vi "Write Solvent Table.vi"(8 "Error In":errorcluster, 10 "Layer Information Array In":T1 {"Deposition Method" items=["Front Electrode", "Electron Transport Layer", "Active Layer", "Hole Transport Layer", "Back Electrode", "Custom Layer"]; "Layer Type" items=["Front Electrode", "Electron Transport Layer", "Active Layer", "Hole Transport Layer", "Back Electrode", "Custom Layer"]}, 11 "Database Full Information In":T2 {"Database Write Information"."Layer Information Array"."Deposition Method" items=["Blade Coating", "Spin Coating", "Thermal Evaporation", "E-Beam Evaporation", "Sputtering", "Drop Casting", "Dip Coating", "Pulsed Laser Deposition", "Chemival Vapour Deposition", "Atomic Layer Deposition", "Spray Coating", "Screen Printing", "Electroplating", "Molecular Beam Epitaxy", "Custom Deposition"]; "Database Write Information"."Layer Information Array"."Layer Type" items=["Front Electrode", "Electron Transport Layer", "Active Layer", "Hole Transport Layer", "Back Electrode", "Custom Layer"]}) -> (0 "Error Out":errorcluster, 3 "Database Full Information Out":T2 {"Database Write Information"."Layer Information Array"."Deposition Method" items=["Blade Coating", "Spin Coating", "Thermal Evaporation", "E-Beam Evaporation", "Sputtering", "Drop Casting", "Dip Coating", "Pulsed Laser Deposition", "Chemival Vapour Deposition", "Atomic Layer Deposition", "Spray Coating", "Screen Printing", "Electroplating", "Molecular Beam Epitaxy", "Custom Deposition"]; "Database Write Information"."Layer Information Array"."Layer Type" items=["Front Electrode", "Electron Transport Layer", "Active Layer", "Hole Transport Layer", "Back Electrode", "Custom Layer"]})   [LabVIEW 2020]
uses:
  Data Clusters/Database Information.ctl
  Data Clusters/Layer Information Cluster.ctl
  <vilib>/addons/database/Connection.llb/Conn ObjectReference.ctl
  <vilib>/addons/database/NI_Database_API.lvlib
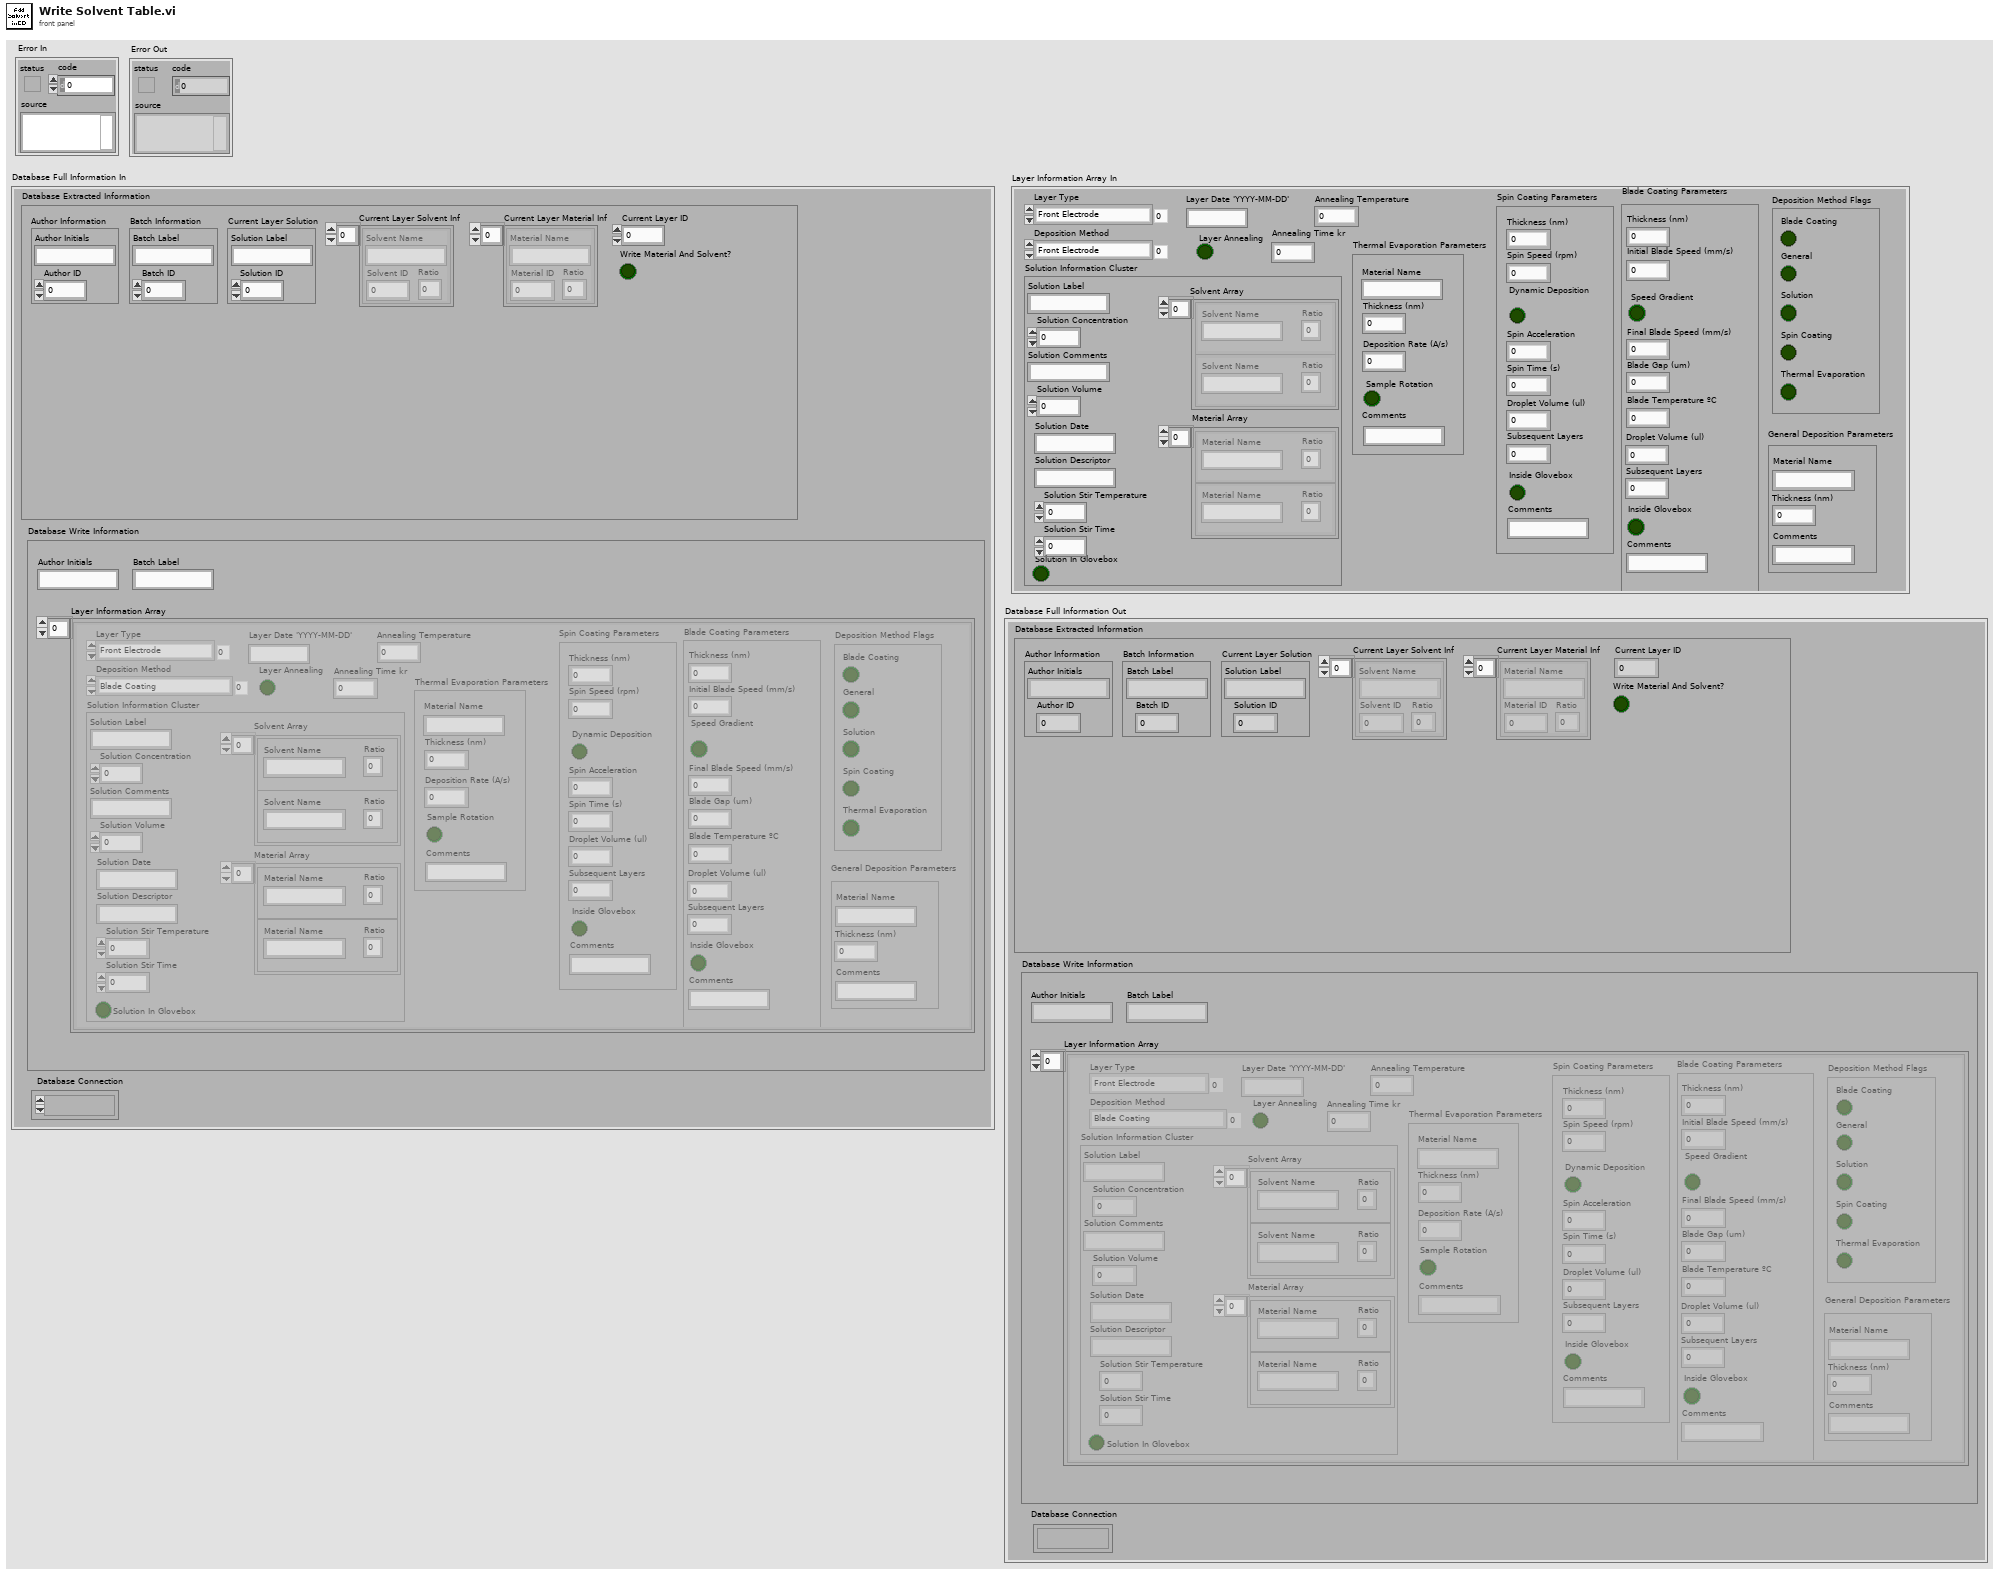
[diagram p1: front panel]
types:
  T1 = typedef "Layer Information Cluster.ctl" = cluster{"Solution Information Cluster":cluster{"Solution Label":string, "Solution Concentration":dbl, "Solution Comments ":string, "Solution Volume ":dbl, "Solution Date ":string, "Solution Descriptor ":string, "Solution Stir Temperature ":dbl, "Solution Stir Time ":dbl, "Solution In Glovebox":bool, "Solvent Array":cluster{"Solvent Name":string, "Ratio":dbl}[], "Material Array":cluster{"Material Name":string, "Ratio":dbl}[]}, "Layer Type":u16, "Deposition Method":u16, "Layer Annealing":bool, "General Deposition Parameters":cluster{"Thickness (nm)":dbl, "Comments":string, "Material Name":string}, "Blade Coating Parameters":cluster{"Thickness (nm)":dbl, "Initial Blade Speed (mm/s)":dbl, "Speed Gradient":bool, "Final Blade Speed (mm/s)":dbl, "Blade Gap (um)":dbl, "Droplet Volume (ul)":dbl, "Subsequent Layers":dbl, "Inside Glovebox":bool, "Comments":string, "Blade Temperature ºC":dbl}, "Spin Coating Parameters":cluster{"Thickness (nm)":dbl, "Spin Speed (rpm)":dbl, "Dynamic Deposition":bool, "Spin Acceleration":dbl, "Spin Time (s)":dbl, "Droplet Volume (ul)":dbl, "Subsequent Layers":dbl, "Inside Glovebox":bool, "Comments":string}, "Thermal Evaporation Parameters":cluster{"Deposition Rate (A/s)":dbl, "Thickness (nm)":dbl, "Comments":string, "Material Name":string, "Sample Rotation":bool}, "Layer Date 'YYYY-MM-DD'":string, "Annealing Time kr":dbl, "Annealing Temperature":dbl, "Deposition Method Flags":cluster{"Blade Coating":bool, "General ":bool, "Solution":bool, "Spin Coating":bool, "Thermal Evaporation":bool}}
  T2 = typedef "Database Information.ctl" = cluster{"Database Extracted Information":cluster{"Author Information":cluster{"Author Initials":string, "Author ID":i32}, "Batch Information":cluster{"Batch Label":string, "Batch ID":i32}, "Current Layer Solution":cluster{"Solution Label":string, "Solution ID":i32}, "Current Layer ID":i32, "Current Layer Solvent Inf":cluster{"Solvent Name":string, "Solvent ID":i32, "Ratio":dbl}[], "Current Layer Material Inf":cluster{"Material Name":string, "Material ID":i32, "Ratio":dbl}[], "Write Material And Solvent?":bool}, "Database Write Information":cluster{"Author Initials":string, "Batch Label":string, "Layer Information Array":T1[]}, "Database Connection":T3}
  T3 = typedef "NI_Database_API.lvlib/Conn ObjectReference.ctl" = refnum<k1>
  T4 = cluster{"Solvent Name":string, "Solvent ID":i32, "Ratio":dbl}
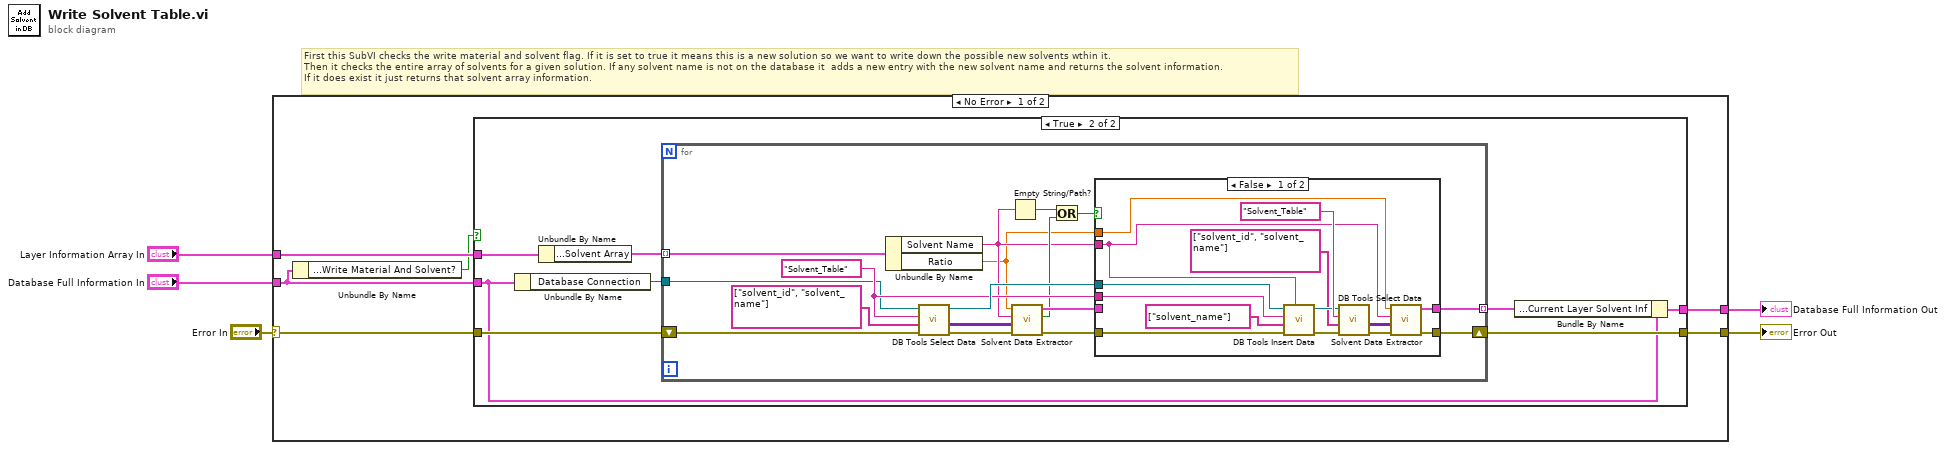
[diagram p0: block diagram]
diagram:
  # "First this SubVI checks the write material and solvent flag. If it is set to true it means this is a new solution so we want to write down the possible new solvents wthin it.\nThen it checks the entire array of solvents for a given solution. If any solvent name is not on the database it  adds a new entry with the new solvent name and returns the solvent information.\nIf it does exist it just returns that solvent array information."
  n1 = case shown="No Error" "Error In" {
    selector: "Error In" -> [w11 w56]
    tunnel: [w10 w56] -> w3
    tunnel: "Database Full Information In" -> [w7 w55]
    tunnel: [w9 w55] -> w2
    tunnel: "Layer Information Array In" -> [w8 _]
    frame No Error {
      n2 = Unbundle By Name(w7) -> ("Database Extracted Information.Write Material And Solvent?"=w6:bool)
      n3 = case shown="True" w6 {
        tunnel: w11 -> [w12 w21]
        tunnel: [w12 w20] -> w10
        tunnel: w7 -> [w13 w19]
        tunnel: [w13 w17] -> w9
        tunnel: w8 -> [_ w15]
        frame False {
        }
        frame True {
          n4 = Unbundle By Name(w19) -> ("Database Connection"=w16:T3)
          n5 = Unbundle By Name(w15) -> ("Solution Information Cluster.Solvent Array"=w14:cluster{"Solvent Name":string, "Ratio":dbl}[])
          n6 = for {
            tunnel: w14 -> [w24] mode=indexing
            tunnel: [w31] -> w18 mode=indexing
            tunnel: w16 -> [w30]
            shift-right: [w34] -> w20
            shift-left: w21 -> [w35]
            w36 = "Solvent_Table" ("table")
            n7 = Unbundle By Name(w24) -> ("Solvent Name"=w23:string, "Ratio"=w22:dbl)
            n8 = call <vilib>:"DB Tools Select Data.vi"("error in (no error)"=w35, "columns"=string[] ["solvent_id", "solvent_name"], "table"=w36, "connection reference"=w30) -> ("error out"=w29:errorcluster, "data"=w28:variant[][], "connection reference out"=w38:T3)  [unwired: 2 in]
            n9 = Empty String/Path?(string/path=w23) -> (empty?=w32:bool)
            n10 = call "Solvent Data Extractor.vi"("Error In"=w29, "Solvent Data"=w28, "Solvent Name"=w23, "Ratio"=w22) -> ("Error Out"=w25:errorcluster, "Exists?"=w26:bool, "Solvent Information"=w27:T4)  [unwired: 5 in]
            n11 = Or(x=w32, y=w26) -> (x .or. y?=w33:bool)
            n12 = case shown="False" w33 {
              tunnel: w23 -> [w42 _]
              tunnel: w25 -> [w52 w54]
              tunnel: w38 -> [w51 _]
              tunnel: w36 -> [w50 _]
              tunnel: [w40 w54] -> w34
              tunnel: w27 -> [_ w53]
              tunnel: [w41 w53] -> w31
              tunnel: w22 -> [w39 _]
              frame False {
                n13 = call <vilib>:"DB Tools Insert Data.vi"("data"=w42, "error in (no error)"=w52, "columns"=string[] ["solvent_name"], "table"=w50, "connection reference"=w51) -> ("error out"=w44:errorcluster, "connection reference out"=w47:T3)  [unwired: 5 in]
                n14 = call <vilib>:"DB Tools Select Data.vi"("error in (no error)"=w44, "columns"=string[] ["solvent_id", "solvent_name"], "table"="Solvent_Table", "connection reference"=w47) -> ("error out"=w43:errorcluster, "data"=w45:variant[][])  [unwired: 2 in, 1 out]
                n15 = call "Solvent Data Extractor.vi"("Error In"=w43, "Solvent Data"=w45, "Solvent Name"=w42, "Ratio"=w39) -> ("Error Out"=w40:errorcluster, "Solvent Information"=w41:T4)  [unwired: 5 in, 1 out]
              }
              frame True {
              }
            }
          }
          n16 = Bundle By Name(cluster=w19, "Database Extracted Information.Current Layer Solvent Inf"=w18) -> (w17:T2)
        }
      }
    }
    frame Error {
    }
  }
  "Error Out" <- w3
  "Database Full Information Out" <- w2
